vi "PKG_IMC_PWMpropFollowEX.vi"(0 "handle":u32, 1 "PWMend":dbl, 2 "ch":i32, 3 "tgEnd":dbl, 5 "polar":i32, 7 "freq":dbl, 9 "PWMstart":dbl, 12 "offset":dbl, 13 "tgStart":dbl, 14 "tgid":i32) -> (4 "handle out":u32, 6 "function return":i32)   [LabVIEW 2011, in "IMC_Pkg4xxx.lvlib"]
doc: "PKG_IMC_PWMpropFollowEX(IMC_HANDLE handle, int polar, double freq, double PWMstart, double PWMend, double offset, int ch, double tgStart, double tgEnd, int tgid);"
uses:
  IMC_Pkg4xxx.lvlib
  IMC_Pkg4xxx.dll
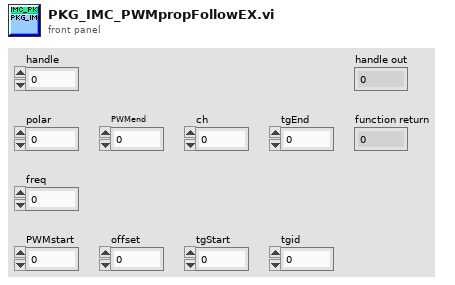
[diagram p1: front panel]
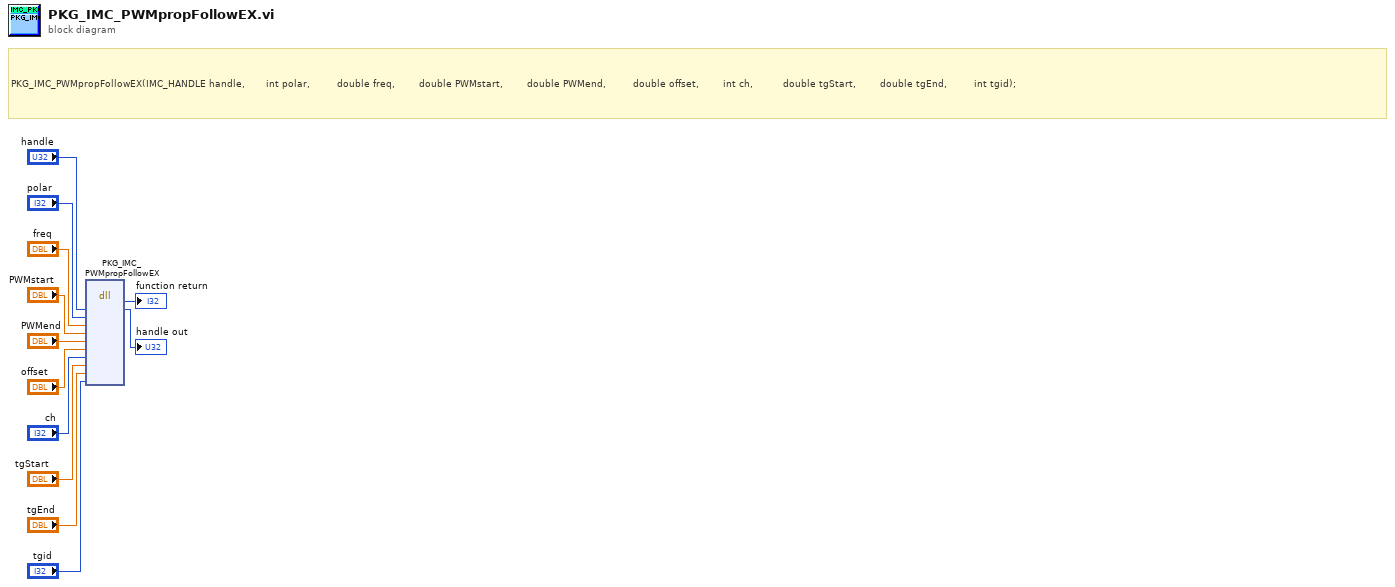
[diagram p0: block diagram]
diagram:
  # "PKG_IMC_PWMpropFollowEX(IMC_HANDLE handle, \t\t\t\t\t\tint polar,\t\t\t\t\t\t\t\t\tdouble freq,\t\t\t\t\t\t\t\tdouble PWMstart, \t\t\t\t\t\t\tdouble PWMend, \t\t\t\t\t\t\t\tdouble offset,\t\t\t\t\t\t\t\tint ch,\t\t\t\t\t\t\t\t\t\tdouble tgStart, \t\t\t\t\t\t\tdouble tgEnd, \t\t\t\t\t\t\t\tint tgid);"
  n1 = dll-call lib="PTH1mabs F光盘刻录\niMC MotionIMCNet_V4.0IMCAppincLabviewIMC_PKG4xxxIMC_PKG4xxx\nIMC_Pkg4xxx.*" fn="PKG_IMC_PWMpropFollowEX"("handle"="handle", "polar"="polar", "freq"="freq", "PWMstart"="PWMstart", "PWMend"="PWMend", "offset"="offset", "ch"="ch", "tgStart"="tgStart", "tgEnd"="tgEnd", "tgid"="tgid") -> (→"function return":i32, "handle"=→"handle out":u32)  [unwired: 12 in, 2 out]
